vi "To XML (Core).vi"(8 "error in (no error)":errorcluster, 10 "Parent":refnum<k20>, 11 "Serializable in":refnum<class "Serializable.lvclass">) -> (0 "error out":errorcluster)   [LabVIEW 2013, in "JUnit XML.lvlib" / "Serializable.lvclass"]
doc: "Serializes a JUnit object to XML and adds it to the provided <B>parent</B> node.\n\nThe parent node must be an element or document."
uses:
  Serializable.lvclass
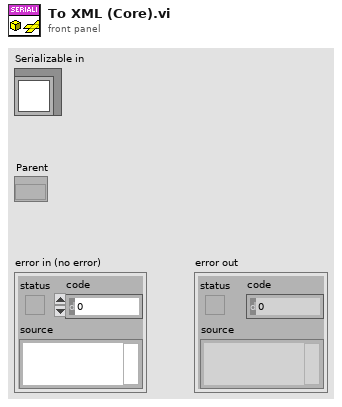
[diagram p1: front panel]
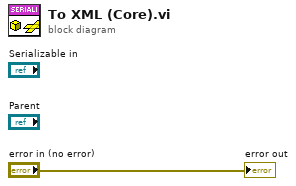
[diagram p0: block diagram]
diagram:
  "error out" <- "error in (no error)"
